vi "BCtr3.vi"() -> ()   [LabVIEW 2015]
panel:
  out "Array 2":dbl[](array[numeric])
  out "String":string
  in  "idx":dbl
  out "error out":errorcluster
  out "OK":bool
  out "ValuesDisp":dbl[][](array[numeric])
  out "Modes":string[](array[string])
  in  "Array":string[](array[string])
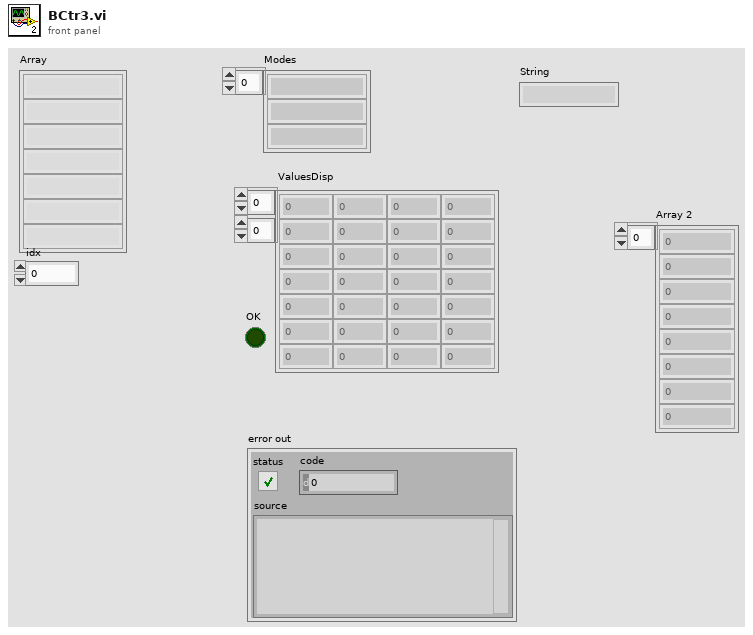
[diagram p1: front panel]
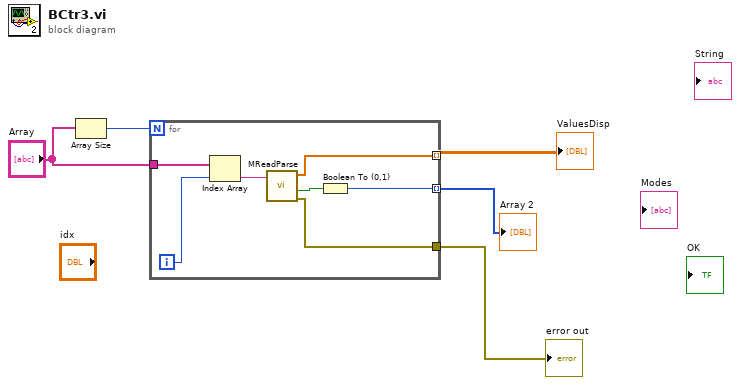
[diagram p0: block diagram]
diagram:
  n1 = Array Size(array="Array") -> (size(s)=w4:i32)
  n2 = for {
    N: w4 -> [_]
    tunnel: "Array" -> [w12]
    tunnel: [w9] -> w3
    tunnel: [w8] -> w2 mode=indexing
    tunnel: [w6] -> w1 mode=indexing
    i -> [w10]
    n3 = Index Array(array=w12, index=w10) -> (element=w11:string)
    n4 = call "MReadParse.vi"("StrIn"=w11) -> ("error out"=w9:errorcluster, "AllAck"=w7:bool, "Values"=w8:dbl[])  [unwired: 7 in, 1 out]
    n5 = Boolean To (0,1)(Boolean=w7) -> (0, 1=w6:i16)
  }
  "ValuesDisp" <- w2
  "error out" <- w3
  "Array 2" <- w1
